vi "sub_getControlReferences.vi"(10 "board label":string, 11 "VI in":refnum<vi>) -> (0 "error out":errorcluster, 3 "Controls[]":refnum<vi>[](array[refnum]))   [LabVIEW 2018]
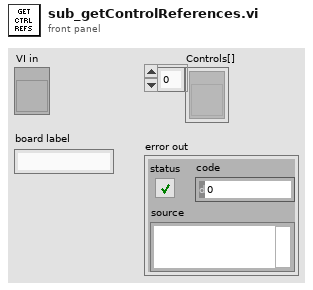
[diagram p1: front panel]
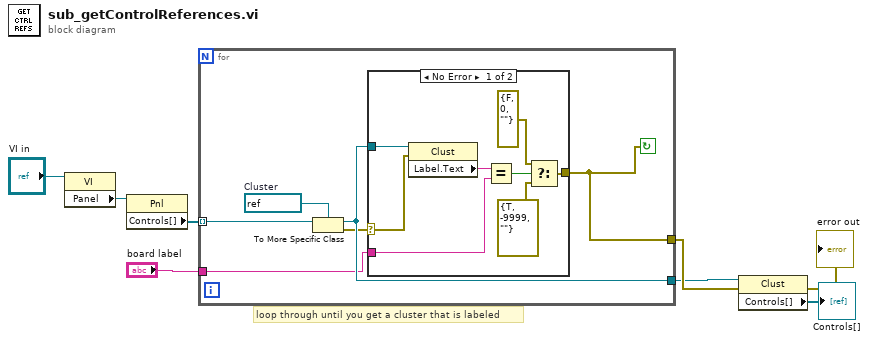
[diagram p0: block diagram]
diagram:
  # "loop through until you get a cluster that is labeled"
  n1 = property class="VI"(reference="VI in") -> ("Panel"=w2:refnum<vi>)  [unwired: 1 in, 2 out]
  n2 = property class="Pnl"(reference=w2) -> ("Controls[]"=w5:refnum<vi>[])  [unwired: 1 in, 2 out]
  n3 = for {
    tunnel: [w12] -> w3
    tunnel: w5 -> [w13] mode=indexing
    tunnel: "board label" -> [w10]
    tunnel: [w9] -> w7
    stop <- w9 continue-if-true
    w14 = refnum<vi> refnum  # Cluster
    n4 = To More Specific Class(target class=w14, reference=w13) -> (specific class reference=w12:refnum<vi>, error out=w11:errorcluster)  [unwired: 1 in]
    n5 = case shown="No Error" w11 {
      selector: w11 -> [w19 w23]
      tunnel: w12 -> [w22 _]
      tunnel: w10 -> [w20 _]
      tunnel: [w15 w23] -> w9
      frame No Error {
        n6 = property class="Clust"(reference=w22, error in=w19) -> ("Label.Text"=w21:string)  [unwired: 2 out]
        n7 = Equal?(x=w21, y=w20) -> (x = y?=w18:bool)
        n8 = Select(t=errorcluster {"status"=FALSE, "code"=0, "source"=""} ("error constant"), s=w18, f=errorcluster {"status"=TRUE, "code"=-9999, "source"=""}) -> (s? t:f=w15:errorcluster)
      }
      frame Error {
      }
    }
  }
  n9 = property class="Clust"(reference=w3, error in=w7) -> (error out=→"error out":errorcluster, "Controls[]"=→"Controls[]":refnum<vi>[])  [unwired: 1 out]
